vi "Noise_measurements.vi"() -> ()   [LabVIEW 2015]
uses:
  <vilib>/express/express analysis/Spectral/Block/exnSpectralBlock spectral measurements power poly.vi
  <vilib>/express/express analysis/Spectral/Block/exnSpectralBlock spectral measurements power WFM.vi
  <vilib>/express/express analysis/Spectral/XNode/ExpressSpectralMeasurementsBlockNode.xnode
panel:
  out "Waveform Graph":cluster{"f0":dbl, "df":dbl, "magnitude":dbl[]}(graph)
  out "IV converter":cluster{dbl[], dbl[]}
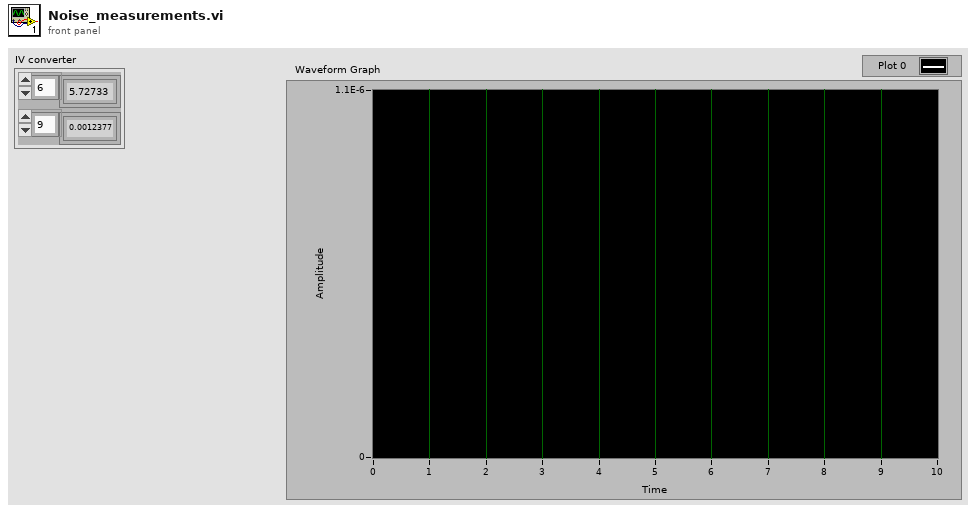
[diagram p1: front panel]
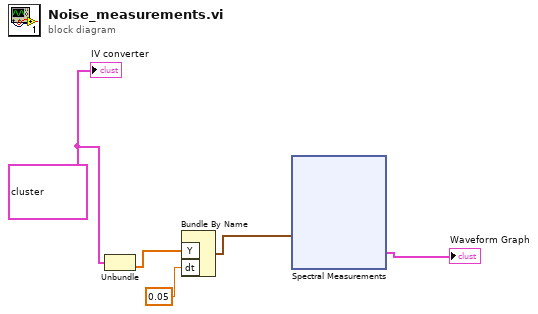
[diagram p0: block diagram]
diagram:
  w5 = cluster{dbl[], dbl[]} {array[2031 elements], array[2031 elements]} ("IV converter")
  n1 = Unbundle(w5) -> (w4:dbl[])  [unwired: 1 out]
  n2 = Bundle By Name("Y"=w4, "dt"=0.05) -> (w3:waveform(dbl))  [unwired: 1 in]
  n3 = xnode "Spectral Measurements"("Signals"=w3) -> ("Power Spectrum"=→"Waveform Graph":cluster{"f0":dbl, "df":dbl, "magnitude":dbl[]})  [unwired: 1 in, 1 out]
  "IV converter" <- w5
